vi "FGV FTP WebDAV.vi"(4 "Connect Timeout (4000 ms)":u32=4000 caption="Verbindungs-Timeout (4000 ms)", 6 "Aktionen":T2, 7 "native Error":bool, 8 "Fehler (Eingang)":errorcluster, 9 "Password":string="iag", 10 "User Name":string="iag", 11 "System Session Ref":refnum<k21>="cRIO-9068 (10.1.128.164)") -> (0 "Fehler (Ausgang)":errorcluster, 1 "WebDAV":bool, 2 "ftp":bool, 3 "ftp webDAV":T1=enum."ftp", 5 "Runtimes":string[](array[string]))   [LabVIEW 2020, in "FTP WebDAV.lvlib"]
uses:
  FTP WebDAV.lvlib
  Aktionen FTP WebDAV.ctl
  Enum FTP WebDAV.ctl
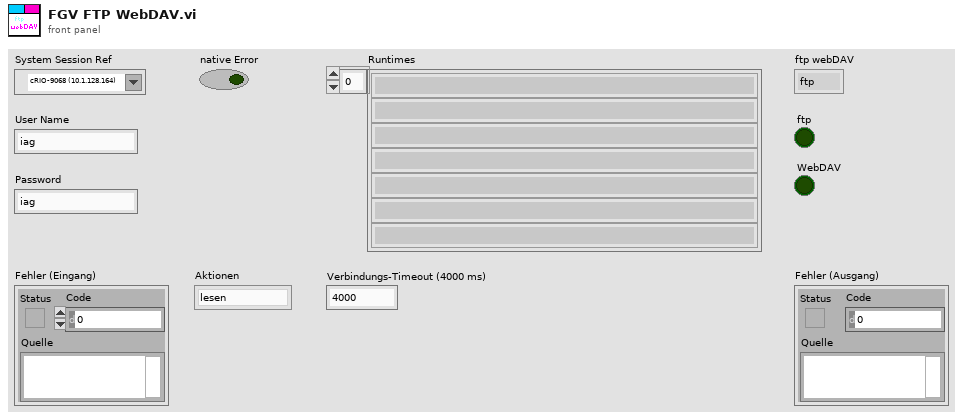
[diagram p1: front panel]
types:
  T1 = typedef "FTP WebDAV.lvlib/Enum FTP WebDAV.ctl" = enum16{" nix", "ftp", "webDAV"}
  T2 = typedef "FTP WebDAV.lvlib/Aktionen FTP WebDAV.ctl" = enum16{"lesen", "erkennen"}
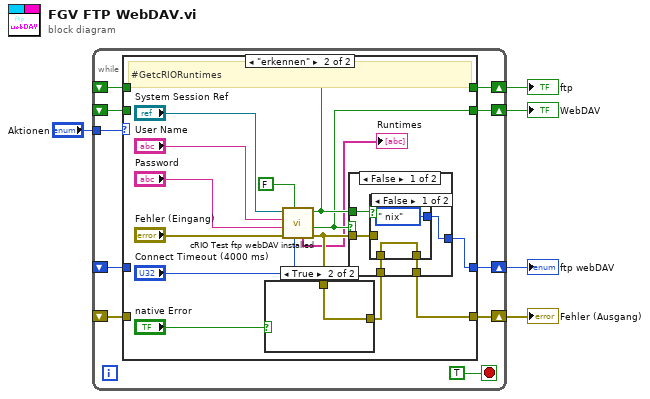
[diagram p0: block diagram]
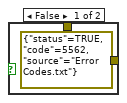
[diagram p3: hidden frame]
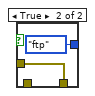
[diagram p4: hidden frame]
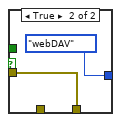
[diagram p5: hidden frame]
diagram:
  n1 = while {
    tunnel: "Aktionen" -> [w14]
    shift-right: [w13] -> w4
    shift-left: _ -> [w12]
    shift-right: [w10] -> w3
    shift-left: _ -> [w11]
    shift-right: [w9] -> w2
    shift-left: _ -> [w8]
    shift-right: [w7] -> w1
    shift-left: _ -> [w6]
    stop <- TRUE stop-if-true
    n2 = case shown="\"erkennen\"" w14 {
      tunnel: [w19 w33] -> w13
      tunnel: w12 -> [w19 _]
      tunnel: w11 -> [w18 _]
      tunnel: [w18 w31] -> w10
      tunnel: [w17 w25] -> w9
      tunnel: w8 -> [w17 _]
      tunnel: [w16 w24] -> w7
      tunnel: w6 -> [w16 _]
      frame "lesen", Default {
      }
      frame "erkennen" {
        # "#GetcRIORuntimes"
        n3 = call "cRIO Test ftp webDAV installed.vi"("Connect Timeout (4000 ms)"="Connect Timeout (4000 ms)", "PC"=FALSE, "error in (no error)"="Fehler (Eingang)", "Password"="Password", "User Name"="User Name", "System Session Ref"="System Session Ref") -> ("error out"=w22:errorcluster, "WebDAV"=w24:bool, "ftp"=w25:bool, "Runtimes"=→"Runtimes":string[])  [unwired: 2 in]
        n4 = case shown="True" "native Error" {
          tunnel: [errorcluster {"status"=TRUE, "code"=5562, "source"="Error Codes.txt"} ("error out") w35] -> w32
          tunnel: w22 -> [_ w35]
          frame False {
          }
          frame True {
          }
        }
        n5 = case shown="False" w24 {
          tunnel: [w39 Enum_FTP_WebDAV."webDAV" ("ftp webDAV")] -> w33
          tunnel: w25 -> [w40 _]
          tunnel: w32 -> [w38 _]
          tunnel: w22 -> [w36 w45]
          tunnel: [w37 w45] -> w31
          frame False {
            n6 = case shown="False" w40 {
              tunnel: [Enum_FTP_WebDAV." nix" ("ftp webDAV") Enum_FTP_WebDAV."ftp" ("ftp webDAV")] -> w39
              tunnel: w38 -> [w41 _]
              tunnel: [w41 w43] -> w37
              tunnel: w36 -> [_ w43]
              frame False {
              }
              frame True {
              }
            }
          }
          frame True {
          }
        }
      }
    }
  }
  "Fehler (Ausgang)" <- w3
  "ftp webDAV" <- w4
  "WebDAV" <- w1
  "ftp" <- w2
